vi "Send Finish.vi"(8 "Error in":errorcluster, 10 "Actor":refnum<class "Actor.lvclass">) -> ()   [LabVIEW 2025, in "jettl.lvlib" / "Actor.lvlib"]
uses:
  Actor.lvlib
  Finish Msg/Finish Msg.lvlib
  Actor/Actor.lvclass
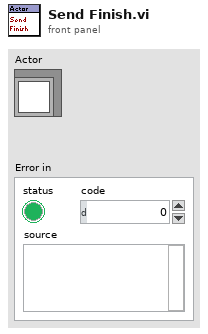
[diagram p1: front panel]
types:
  T1 = typedef "jettl.lvlib/Actor.lvlib/Created Aliases.ctl" = set{string}
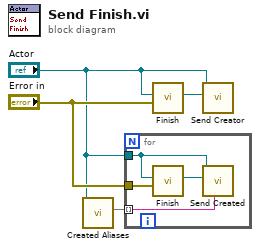
[diagram p0: block diagram]
diagram:
  n1 = call-dynamic "Created Aliases.vi"("Actor in"="Actor") -> ("Created Aliases"=w4:T1)  [unwired: 10 in]
  n2 = for {
    tunnel: "Actor" -> [w8]
    tunnel: w4 -> [w5] mode=indexing
    tunnel: "Error in" -> [w6]
    n3 = call "Finish.vi"("Error"=w6, "Actor"=w8) -> ("Msg"=w7:refnum<class "Msg.lvclass">)  [unwired: 9 in]
    n4 = call-dynamic "Send Created.vi"("Alias"=w5, "Msg"=w7, "Actor in"=w8) -> ()  [unwired: 8 in, 1 out]
  }
  n5 = call "Finish.vi"("Error"="Error in", "Actor"="Actor") -> ("Msg"=w3:refnum<class "Msg.lvclass">)  [unwired: 9 in]
  n6 = call-dynamic "Send Creator.vi"("Msg"=w3, "Actor in"="Actor") -> ()  [unwired: 9 in, 1 out]
